vi "uTTA_Read_File_UI.vi"() -> ()   [LabVIEW 2021]
panel:
  out "Connected":bool
  in  "Delete":bool
  out "Last Line":string
  in  "EXIT":bool
  in  "File":u16(ring)
  in  "Connect":bool
  in  "Read":bool
  out "RunTime":dbl format="%ds"
  out "Read took":i32 format="%.0fms"
  out "Timeout Expanded":bool
  out "Received":string
  out "error out":errorcluster
  in  "VISA resource name":refnum<visa-resource-name>
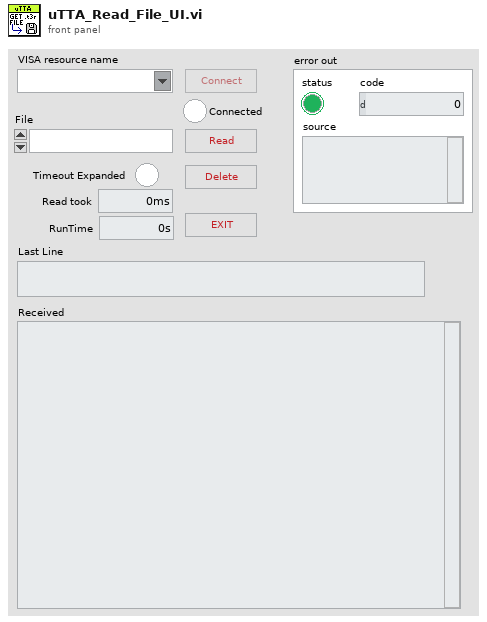
[diagram p1: front panel]
types:
  T1 = enum8{"Enabled", "Disabled", "Disabled and Grayed Out"}
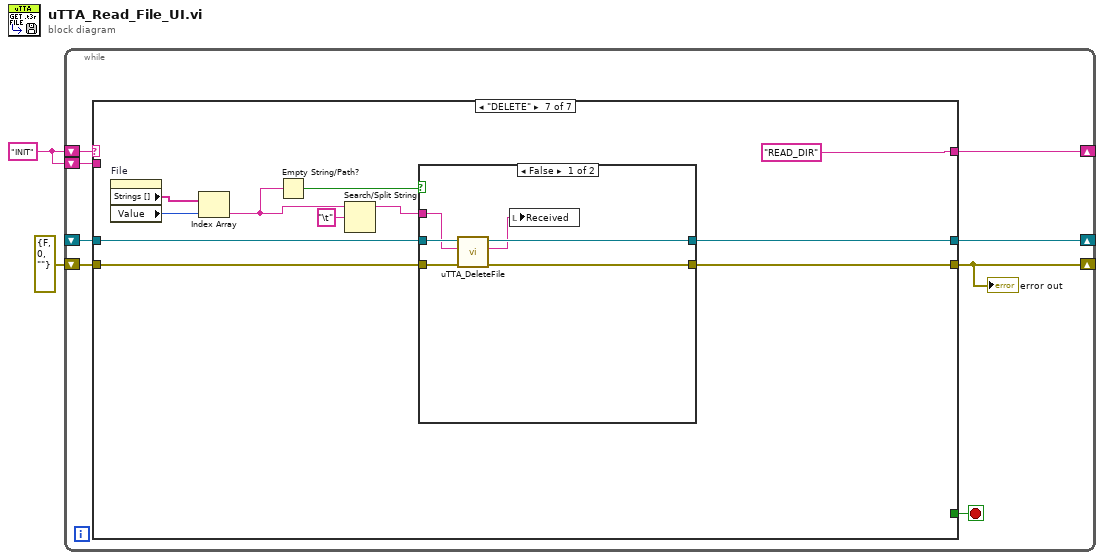
[diagram p0: block diagram]
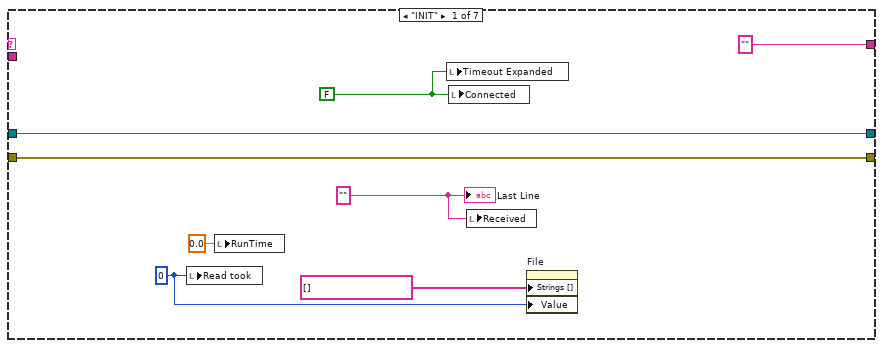
[diagram p2: hidden frame]
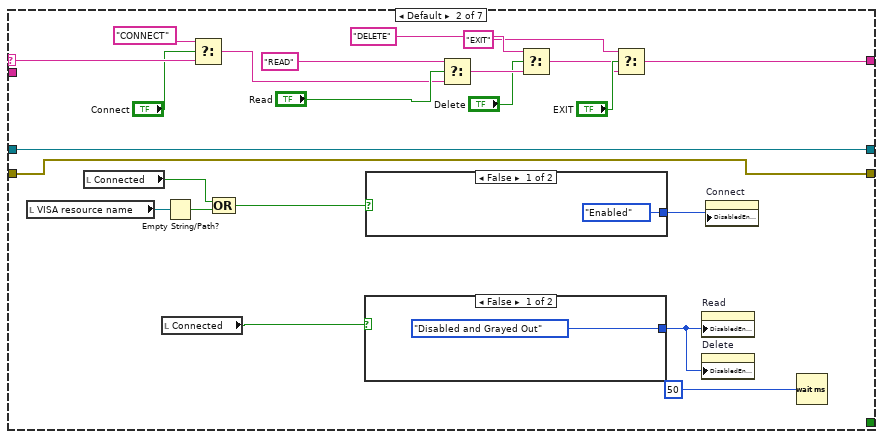
[diagram p3: hidden frame]
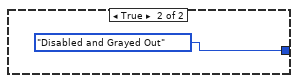
[diagram p4: hidden frame]
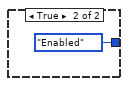
[diagram p5: hidden frame]
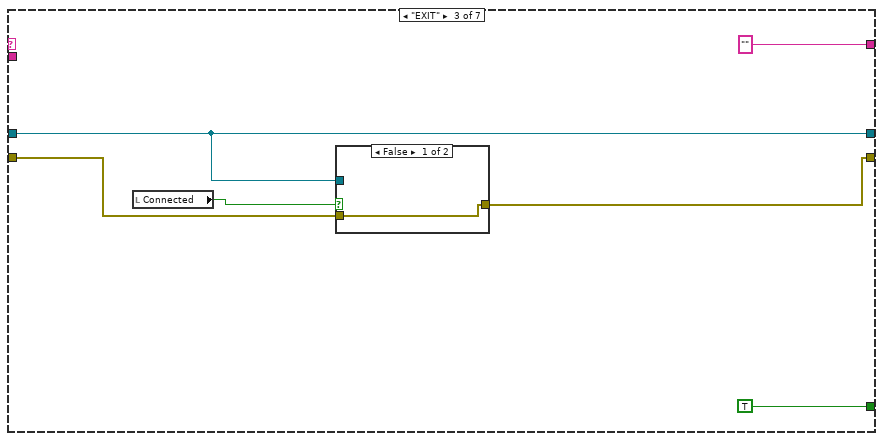
[diagram p6: hidden frame]
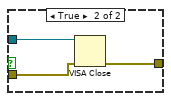
[diagram p7: hidden frame]
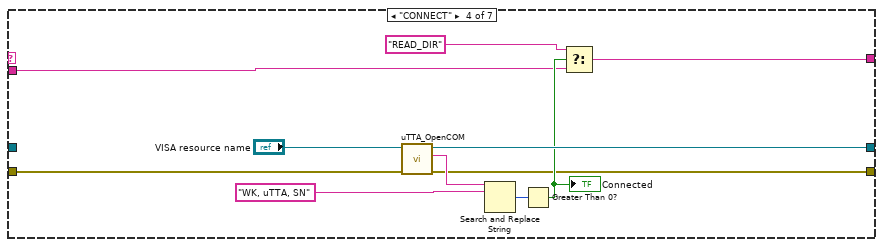
[diagram p8: hidden frame]
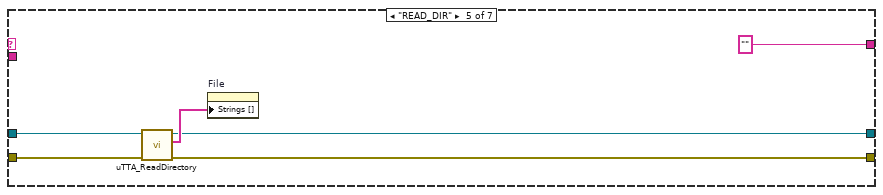
[diagram p9: hidden frame]
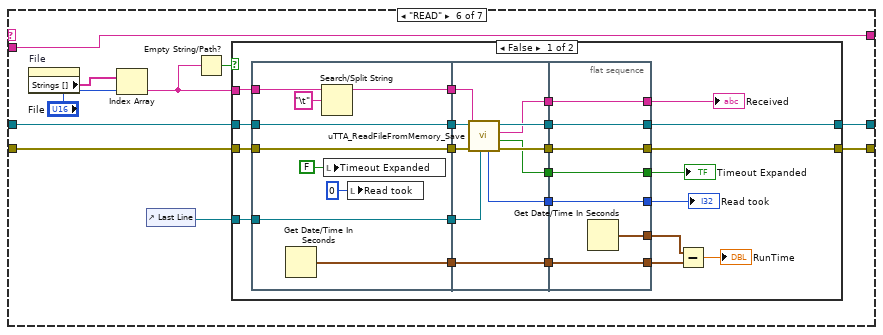
[diagram p10: hidden frame]
diagram:
  w1 = "INIT" ("Filename")
  n1 = while {
    shift-right: [w8] -> _
    shift-left: w1 -> [w9]
    shift-right: [w7] -> _
    shift-left: _ -> [w6]
    shift-left: w1 -> [w5]
    shift-right: [w3] -> _
    shift-left: errorcluster {"status"=FALSE, "code"=0, "source"=""} ("error out") -> [w4]
    stop <- w10 stop-if-true
    n2 = case shown="\"DELETE\"" w9 {
      selector: w9 -> [_ w36 _ _ _ _ _]
      tunnel: [_ _ TRUE ("EXIT") _ _ _ _] -> w10
      tunnel: ["" ("t") w24 "" ("t") w59 "" ("Filename") w75 "READ_DIR" ("t")] -> w8
      tunnel: [w14 w22 w50 w65 w70 w77 w139] -> w7
      tunnel: w6 -> [w14 w22 w50 _ w71 w76 w140]
      tunnel: w5 -> [_ _ _ w58 _ w75 _]
      tunnel: w4 -> [w11 w20 w47 w57 w68 w74 w138]
      tunnel: [w11 w20 w46 w56 w67 w73 w137] -> w3
      frame "INIT" {
        w13 = 0 ("Read took ms")
        w17 = "" ("Last Line")
        w12 = FALSE ("Connected")
        n3 = local write "Read took"(w13) -> ()
        n4 = local write "RunTime"(0.0 ("RunTime")) -> ()
        n5 = local write "Timeout Expanded"(w12) -> ()
        n6 = local write "Connected"(w12) -> ()
        n7 = local write "Received"(w17) -> ()
        n8 = property on="File" class="Ring (strict)"("Strings []"=string[] [], "Value"=w13) -> ()  [unwired: 2 in, 2 out]
        "Last Line" <- w17
      }
      frame Default {
        n9 = local read "VISA resource name"() -> (w39:refnum<visa-resource-name>)
        n10 = local read "Connected"() -> (w21:bool)
        n11 = local read "Connected"() -> (w19:bool)
        n12 = Empty String/Path?(string/path=w39) -> (empty?=w28:bool)
        n13 = Select(t="CONNECT", s="Connect", f=w36) -> (s? t:f=w35:string)
        n14 = Compound Arithmetic op=OR(w21, w28) -> (w27:bool)
        n15 = case shown="False" w19 {
          tunnel: [T1."Disabled and Grayed Out" ("Disabled") T1."Enabled" ("Disabled")] -> w29
          frame False {
          }
          frame True {
          }
        }
        n16 = case shown="False" w27 {
          tunnel: [T1."Enabled" ("Disabled") T1."Disabled and Grayed Out" ("Disabled")] -> w37
          frame False {
          }
          frame True {
          }
        }
        n17 = Select(t="READ" ("Filename"), s="Read", f=w35) -> (s? t:f=w32:string)
        n18 = Select(t="DELETE", s="Delete", f=w32) -> (s? t:f=w25:string)
        n19 = Select(t="EXIT", s="EXIT", f=w25) -> (s? t:f=w24:string)
        n20 = property on="Read" class="Bool"("DisabledEnum"=w29) -> ()  [unwired: 2 in, 2 out]
        n21 = property on="Delete" class="Bool"("DisabledEnum"=w29) -> ()  [unwired: 2 in, 2 out]
        n22 = property on="Connect" class="Bool"("DisabledEnum"=w37) -> ()  [unwired: 2 in, 2 out]
        n23 = Wait (ms)(milliseconds to wait=u32 50) -> ()  [unwired: 1 out]
      }
      frame "EXIT" {
        n24 = local read "Connected"() -> (w48:bool)
        n25 = case shown="False" w48 {
          tunnel: w50 -> [_ w55]
          tunnel: w47 -> [w52 w54]
          tunnel: [w52 w53] -> w46
          frame False {
          }
          frame True {
            n26 = VISA Close(VISA resource name=w55, error in (no error)=w54) -> (error out=w53:errorcluster)
          }
        }
      }
      frame "CONNECT" {
        n27 = call "uTTA_OpenCOM.vi"("error in"=w57, "VISA in"="VISA resource name") -> ("error out"=w56:errorcluster, "Identity"=w63:string, "VISA out"=w65:refnum<visa-resource-name>)  [unwired: 7 in]
        n28 = Search and Replace String(input string=w63, search string="WK, uTTA, SN") -> (number of replacements=w64:i32)  [unwired: 6 in, 3 out]
        n29 = Greater Than 0?(x=w64) -> (x > 0?=w60:bool)
        "Connected" <- w60
        n30 = Select(t="READ_DIR", s=w60, f=w58) -> (s? t:f=w59:string)
      }
      frame "READ_DIR" {
        n31 = call "uTTA_ReadDirectory.vi"("error in"=w68, "VISA Refnum in"=w71) -> ("error out"=w67:errorcluster, "Files"=w72:string[], "VISA Refnum out"=w70:refnum<visa-resource-name>)  [unwired: 7 in]
        n32 = property on="File" class="Ring (strict)"("Strings []"=w72) -> ()  [unwired: 2 in, 2 out]
      }
      frame "READ" {
        n33 = property on="File" class="Ring (strict)"() -> ("Strings []"=w82:string[])  [unwired: 2 in, 2 out]
        n34 = Index Array(array=w82, index="File") -> (element=w79:string)
        n35 = control-ref of="Last Line"() -> (w78:refnum<vi>)
        n36 = Empty String/Path?(string/path=w79) -> (empty?=w80:bool)
        n37 = case shown="False" w80 {
          tunnel: w76 -> [w91 w133]
          tunnel: w79 -> [w90 _]
          tunnel: w78 -> [w89 _]
          tunnel: [w87 w133] -> w77
          tunnel: w74 -> [w86 w132]
          tunnel: [w84 w132] -> w73
          frame False {
            n38 = flat-sequence {
              tunnel: w90 -> [w108]
              tunnel: w91 -> [w114]
              tunnel: [w114] -> w105
              tunnel: [w113] -> w104
              tunnel: w89 -> [w112]
              tunnel: [w112] -> w88
              tunnel: w86 -> [w111]
              tunnel: [w111] -> w85
              tunnel: [w106] -> w83
              tunnel: w105 -> [w124]
              tunnel: [w123] -> w103
              tunnel: [w122] -> w102
              tunnel: [w120] -> w101
              tunnel: [w119] -> w100
              tunnel: [w118] -> w99
              tunnel: [w117] -> w98
              tunnel: w104 -> [w117]
              tunnel: w88 -> [w116]
              tunnel: w85 -> [w115]
              tunnel: w83 -> [w121]
              tunnel: [w127] -> w95
              tunnel: [w128] -> w96
              tunnel: [w129] -> w97
              tunnel: [w130] -> w87
              tunnel: [w131] -> w84
              tunnel: w103 -> [w131]
              tunnel: w102 -> [w130]
              tunnel: w101 -> [w129]
              tunnel: w100 -> [w128]
              tunnel: w99 -> [w127]
              tunnel: [w126] -> w94
              tunnel: w98 -> [w126]
              tunnel: [w125] -> w93
              frame #0 {
                n39 = Get Date/Time In Seconds() -> (seconds since 1Jan1904=w113:timestamp)
                n40 = Search/Split String(string=w108, search string/char (-)="\t") -> (substring before match=w106:string)  [unwired: 1 in, 2 out]
                n41 = local write "Timeout Expanded"(FALSE ("Timeout Expanded")) -> ()
                n42 = local write "Read took"(0 ("Read took")) -> ()
              }
              frame #1 {
                n43 = call "uTTA_ReadFileFromMemory_Save.vi"("Last Line"=w116, "error in"=w115, "Filename"=w121, "VISA Refnum in"=w124) -> ("error out"=w123:errorcluster, "Timeout Expanded"=w119:bool, "Received"=w120:string, "VISA Refnum out"=w122:refnum<visa-resource-name>, "Read took ms"=w118:i32)  [unwired: 3 in]
              }
              frame #2 {
                n44 = Get Date/Time In Seconds() -> (seconds since 1Jan1904=w125:timestamp)
              }
            }
            n45 = Subtract(x=w93, y=w94) -> (x-y=→"RunTime":dbl)
            "Received" <- w97
            "Timeout Expanded" <- w96
            "Read took" <- w95
          }
          frame True {
          }
        }
      }
      frame "DELETE" {
        n46 = property on="File" class="Ring (strict)"() -> ("Strings []"=w141:string[], "Value"=w143:u16)  [unwired: 2 in, 2 out]
        n47 = Index Array(array=w141, index=w143) -> (element=w135:string)
        n48 = Empty String/Path?(string/path=w135) -> (empty?=w142:bool)
        n49 = Search/Split String(string=w135, search string/char (-)="\t") -> (substring before match=w134:string)  [unwired: 1 in, 2 out]
        n50 = case shown="False" w142 {
          tunnel: w134 -> [w149 _]
          tunnel: w140 -> [w150 w152]
          tunnel: [w148 w152] -> w139
          tunnel: w138 -> [w146 w151]
          tunnel: [w145 w151] -> w137
          frame False {
            n51 = call "uTTA_DeleteFile.vi"("error in"=w146, "Directory Name"=w149, "VISA Refnum in"=w150) -> ("error out"=w145:errorcluster, "Received"=w147:string, "VISA Refnum out"=w148:refnum<visa-resource-name>)  [unwired: 6 in]
            n52 = local write "Received"(w147) -> ()
          }
          frame True {
          }
        }
      }
    }
    "error out" <- w3
  }
